vi "SaveNew.vi"(8 "error in (no error)":errorcluster, 10 "Path":path, 11 "Preferences in":refnum<class "SetListPrefs.lvclass">) -> (0 "error out":errorcluster, 2 "Raw XML":string, 3 "Preferences out":refnum<class "SetListPrefs.lvclass">)   [LabVIEW 2013, in "SetListPrefs.lvclass"]
uses:
  SetListPrefs.lvclass
panel:
  # "Leave Path Deafult as EMPTY PATH"
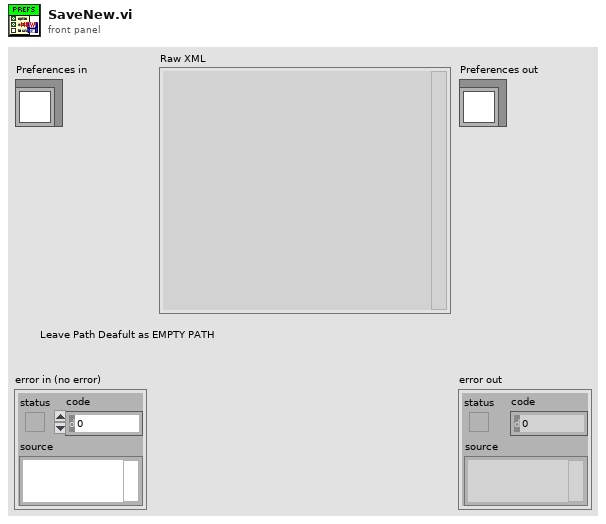
[diagram p1: front panel]
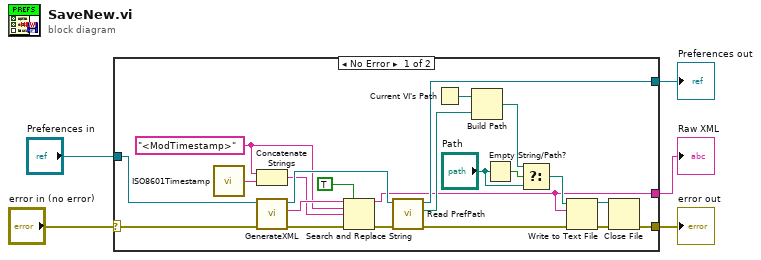
[diagram p0: block diagram]
diagram:
  n1 = case shown="No Error" "error in (no error)" {
    selector: "error in (no error)" -> [w26 w29]
    tunnel: [w20 w29] -> w4
    tunnel: [w19 w28] -> w2
    tunnel: "Preferences in" -> [w27 w28]
    tunnel: [w6 _] -> w1
    frame No Error {
      w9 = "<ModTimestamp>" ("string")
      n2 = call "ISO8601Timestamp.vi"() -> ("ISO8601 Timestamp"=w11:string)
      n3 = Concatenate Strings(w9, w11) -> (w10:string)
      n4 = call "GenerateXML.vi"("error in (no error)"=w26, "Preferences in"=w27) -> ("error out"=w14:errorcluster, "FullXML"=w12:string, "Preferences out"=w13:refnum<class "SetListPrefs.lvclass">)  [unwired: 7 in]
      n5 = Search and Replace String(replace all?=TRUE ("replace all? (F)"), input string=w12, search string=w9, replace string=w10, error in=w14) -> (result string=w6:string, error out=w7:errorcluster)  [unwired: 3 in, 2 out]
      n6 = call-dynamic "Read PrefPath.vi"("error in (no error)"=w7, "Preferences in"=w13) -> ("error out"=w23:errorcluster, "PrefPath"=w24:path, "Preferences out"=w19:refnum<class "SetListPrefs.lvclass">)  [unwired: 7 in]
      n7 = Current VI's Path() -> (path=w25:path)
      n8 = Build Path(base path=w25, name or relative path=w24) -> (appended path=w17:path)
      n9 = Empty String/Path?(string/path="Path") -> (empty?=w18:bool)
      n10 = Select(t=w17, s=w18, f="Path") -> (s? t:f=w15:path)
      n11 = Write to Text File(file (use dialog)=w15, text=w6, error in=w23) -> (refnum out=w21:refnum<file>, error out=w22:errorcluster)  [unwired: 1 in, 1 out]
      n12 = Close File(refnum=w21, error in=w22) -> (error out=w20:errorcluster)  [unwired: 1 out]
    }
    frame Error {
    }
  }
  "error out" <- w4
  "Preferences out" <- w2
  "Raw XML" <- w1
